vi "Digital Close.vi"(8 "Error In":errorcluster, 10 "Digtal Channel":u8[](array[numeric]), 11 "LINX Resource":T1) -> (0 "Error Out":errorcluster, 3 "LINX Resource":T1)   [LabVIEW 2011, in "LVH-LINX.lvlib"]
doc: "Close the specified digital IO channels."
uses:
  LVH-LINX.lvlib
  Private/Type Defs/LINX Ref.ctl
  Private/Type Defs/Platform.ctl
  Private/Type Defs/Interface.ctl
  Private/Device/Type Defs/LINX Device Config.ctl
  Private/Device/Type Defs/TCP Config.ctl
  Private/Type Defs/Device Family.ctl
  Private/Type Defs/Peripheral.ctl
  Private/myRIO/myRIO.lvlib
  Private/Device/Device.lvlib
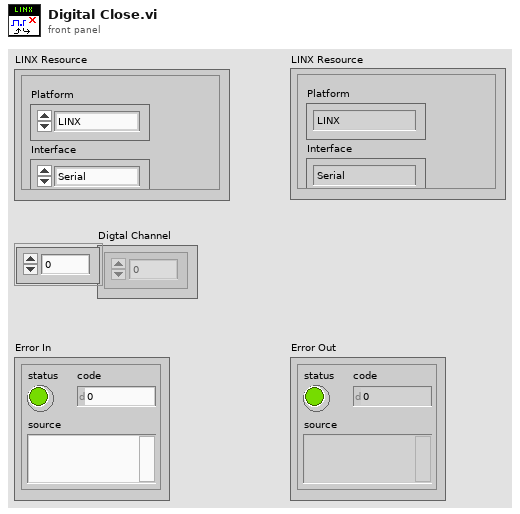
[diagram p1: front panel]
types:
  T1 = typedef "LVH-LINX.lvlib/LINX Ref.ctl" = cluster{"Platform":T2, "Interface":T3, "LINX Device Config":T4}
  T2 = typedef "LVH-LINX.lvlib/Platform.ctl" = enum16{"LINX", "myRIO"}
  T3 = typedef "LVH-LINX.lvlib/Interface.ctl" = enum16{"Serial", "TCP"}
  T4 = typedef "LVH-LINX.lvlib/Device.lvlib/LINX Device Config.ctl" = cluster{"Interface":T3, "COM Port":refnum<visa-resource-name>, "TCP Configuration":T5, "Device Family":T6, "Device ID":u8, "Device Name":string, "TCP Ref":refnum<k5>}
  T5 = typedef "LVH-LINX.lvlib/Device.lvlib/TCP Config.ctl" = cluster{"IP Address":string, "Port":u16}
  T6 = typedef "LVH-LINX.lvlib/Device Family.ctl" = enum8{"National Instruments", "Digilent", "Arduino"}
  T7 = typedef "LVH-LINX.lvlib/Peripheral.ctl" = enum8{"DI", "DO", "AI", "AO", "PWM", "QE", "UART", "I2C", "SPI", "CAN"}
  T8 = typedef "DIO.lvlib/DIO Reference.ctl" = cluster{"myRIO Reference":T9, "DIO Channels List":T13}
  T9 = typedef "myRIO Generic Hardware Reference.ctl" = cluster{"myRIO Model":T10, "myRIO Hardware Reference":T11}
  T10 = typedef "Hardware Version Enum.ctl" = enum16{"Unknown", "myRIO-1900", "myRIO-1950"}
  T11 = typedef "myRIO v1.0 Reference.ctl" = cluster{"Generic FPGA Reference":T12, "Allow multiple opens":bool}
  T12 = typedef "Generic FPGA Reference.ctl" = refnum<k20>
  T13 = typedef "DIO Channels List.ctl" = T14[]
  T14 = typedef "DIO Channels Enum.ctl" = enum16{"Not Connected", "C/DIO0", "C/DIO1", "C/DIO2", "C/DIO3", "C/DIO4", "C/DIO5", "C/DIO6", "C/DIO7", "A/DIO0", "A/DIO1", "A/DIO2", "A/DIO3", "A/DIO4", "A/DIO5", "A/DIO6", "A/DIO7", "A/DIO8", "A/DIO9", "A/DIO10", "A/DIO11", "A/DIO12", "A/DIO13", "A/DIO14", "A/DIO15", "B/DIO0", "B/DIO1", "B/DIO2", "B/DIO3", "B/DIO4", "B/DIO5", "B/DIO6", "B/DIO7", "B/DIO8", "B/DIO9", "B/DIO10", "B/DIO11", "B/DIO12", "B/DIO13", "B/DIO14", "B/DIO15", "LED0", "LED1", "LED2", "LED3", "Button0"}
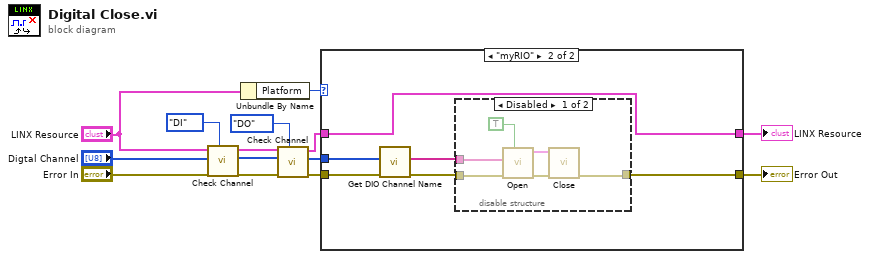
[diagram p0: block diagram]
diagram:
  n1 = call "Check Channel.vi"("Peripheral"=Peripheral."DI", "Error In"="Error In", "Channels"="Digtal Channel", "LINX Resource"="LINX Resource") -> ("Error Out"=w4:errorcluster, "Channels"=w5:u8[], "LINX Resource"=w3:T1)  [unwired: 5 in]
  n2 = Unbundle By Name("LINX Resource") -> ("Platform"=w14:T2)
  n3 = call "Check Channel.vi"("Peripheral"=Peripheral."DO", "Error In"=w4, "Channels"=w5, "LINX Resource"=w3) -> ("Error Out"=w9:errorcluster, "Channels"=w10:u8[], "LINX Resource"=w1:T1)  [unwired: 5 in]
  n4 = case shown="\"myRIO\"" w14 {
    tunnel: w9 -> [w16 w21]
    tunnel: [w16 w18] -> w13
    tunnel: w10 -> [_ w22]
    tunnel: [w15 w17] -> w12
    tunnel: w1 -> [w15 w17]
    frame "LINX", Default {
      # "!!! Send Close Command (Some LINX Devices Might Have A Use For This)"
    }
    frame "myRIO" {
      n5 = call "Get DIO Channel Name.vi"("Error In"=w21, "DIO Channel Nums"=w22) -> ("Error Out"=w19:errorcluster, "DIO Channels"=w20:string[])  [unwired: 8 in]
      n6 = disable-structure shown="Disabled" {
        disable-tunnel: w20 -> [w25 _]
        disable-tunnel: w19 -> [w24 w29]
        disable-tunnel: [w23 w29] -> w18
        frame Disabled {
          n7 = call <vilib>:"Open.vi"("Allow multiple opens?"=TRUE, "error in (no error)"=w24, "Channel Names"=w25) -> ("error out"=w28:errorcluster, "DIO Ref Out"=w27:T8)  [unwired: 7 in]
          n8 = call <vilib>:"Close.vi"("error in (no error)"=w28, "DIO Ref In"=w27) -> ("error out"=w23:errorcluster)  [unwired: 9 in]
        }
        frame Enabled {
          # "myRIO Support Not Installed"
        }
      }
    }
  }
  "Error Out" <- w13
  "LINX Resource" <- w12
